vi "SMTP Email Send Text Message.vi"(0 "smtp session":T1, 2 "return address":string, 3 "character set":string, 5 "recipients":string[](array[string]), 7 "subject":string, 9 "message":string, 11 "error in (no error)":errorcluster, 12 "translit":string) -> (4 "smtp session out":T1, 6 "invalid recipients":string[](array[string]), 15 "error out":errorcluster)   [LabVIEW 2011, in "NewNI_SMTPEmail.lvlib"]
doc: "E-mails the Textual Message to the Recipients using Mailserver.\n\nTextual Message: Textual message to be sent; if empty then the attachments only will be sent.\n\nMailserver: SMTP mailserver to be used to send the mail. Must be either specified here, or setup by using SMTP Setup.vi\n\nReturn Address: your desired return address; can be either specified here, or setup by using SMTP Setup.vi\n\nRecipients: list of mailboxes which specifiy where you want your e-mail sent.\n\nSubject: Subject of your message. Defaults to the string \"None\" if unwired.\n\nCharacter Set: the mailer provides international support. Character set value is intended for use with the foreign (non-US) character sets.\n\nInvalid Recipients: The list of recipients (out of the specified) that do not exist according to the mailserver (may not contain all the invalid recipients, especially if they are nonlocal to the SMTP server)."
uses:
  NewNI_SMTPEmail.lvlib
  SMTP Email Session.ctl
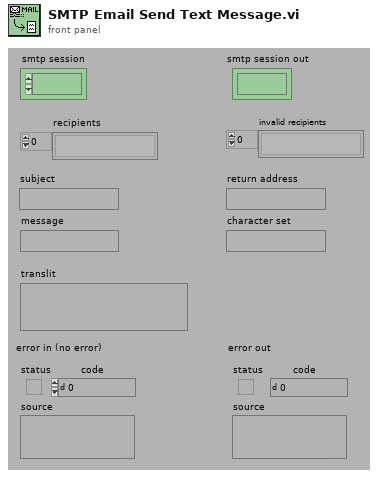
[diagram p1: front panel]
types:
  T1 = typedef "NewNI_SMTPEmail.lvlib/SMTP Email Session.ctl" = refnum<k1>
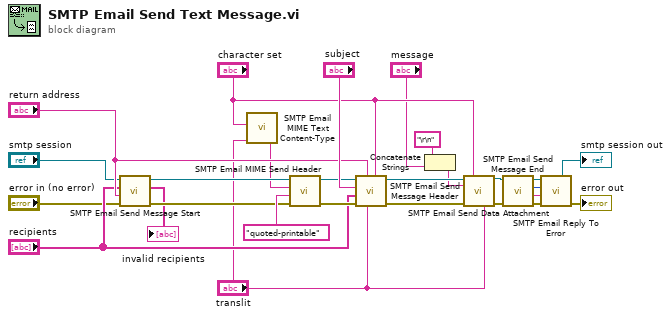
[diagram p0: block diagram]
diagram:
  n1 = call "SMTP Email Send Message Start.vi"("error in (no error)"="error in (no error)", "return address"="return address", "recipients"="recipients", "smtp session"="smtp session") -> ("error out"=w16:errorcluster, "invalid recipients"=→"invalid recipients":string[], "smtp session out"=w15:T1)  [unwired: 1 out]
  n2 = call "SMTP Email MIME Text Content-Type.vi"("translit"="translit", "character set"="character set") -> ("MIME content-type"=w2:string)  [unwired: 1 in, 4 out]
  n3 = call "SMTP Email MIME Send Header.vi"("error in (no error)"=w16, "MIME content-transfer-encoding (7bit)"="quoted-printable" ("Content-Transfer-Encoding (\"7bit\")"), "MIME content-type (multipart/mixed)"=w2, "smtp session"=w15) -> ("error out"=w21:errorcluster, "smtp session out"=w22:T1)  [unwired: 2 out]
  n4 = call "SMTP Email Send Message Header.vi"("character set"="character set", "translit"="translit", "return address"="return address", "error in (no error)"=w21, "recipients"="recipients", "subject"="subject", "smtp session"=w22) -> ("error out"=w23:errorcluster, "smtp session out"=w24:T1)  [unwired: 3 out]
  n5 = Concatenate Strings("\r\n" ("Substring"), "message") -> (w4:string)
  n6 = call "SMTP Email Send Data Attachment.vi"("smtp session"=w24, "character set"="character set", "data"=w4, "error in (no error)"=w23, "translit"="translit") -> ("smtp session out"=w27:T1, "error out"=w26:errorcluster)  [unwired: 1 in, 8 out]
  n7 = call "SMTP Email Send Message End.vi"("error in (no error)"=w26, "smtp session"=w27) -> ("error out"=w11:errorcluster, "reply"=w6:string, "reply code"=w7:i32, "smtp session out"=w10:T1)  [unwired: 1 in, 1 out]
  n8 = call "SMTP Email Reply To Error.vi"("error in (no error)"=w11, "reply string in"=w6, "reply code in"=w7, "smtp session"=w10) -> ("error out"=→"error out":errorcluster, "smtp session out"=→"smtp session out":T1)  [unwired: 2 out]
